vi "Init.vi"(8 "error in (no error)":errorcluster, 11 "BounceTarget in":refnum<class "BounceTarget.lvclass">) -> (0 "error out":errorcluster, 3 "BounceTarget out":refnum<class "BounceTarget.lvclass">)   [LabVIEW 2019, in "RT_Game.lvlib" / "BounceTarget.lvclass"]
uses:
  BounceTarget.lvclass
  BounceTarget.lvclass/BounceTarget.ctl
  GameObject/GameObject.lvclass
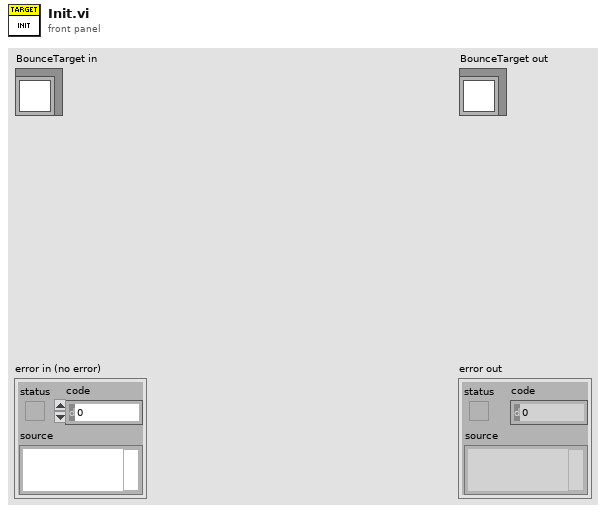
[diagram p1: front panel]
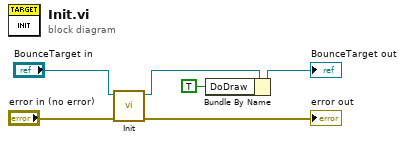
[diagram p0: block diagram]
diagram:
  n1 = call-parent "Init.vi"("error in (no error)"="error in (no error)", "GameObject in"="BounceTarget in") -> ("error out"=→"error out":errorcluster, "GameObject out"=w3:refnum<class "BounceTarget.lvclass">)  [unwired: 8 in]
  n2 = Bundle By Name(cluster=w3, "DoDraw"=TRUE) -> (→"BounceTarget out":refnum<class "BounceTarget.lvclass">)
